vi "Destroy.vi"   [LabVIEW 2018, in "Toolkit.lvlib" / "Agent Identity.lvclass"]
doc: "Deallocates, or frees, the memory allocated for the agent identity object. After this is called, the object can no longer be used in the application without causing a segmentation fault, i.e. crashing LabVIEW. This VI must be called to avoid leaking memory or running out of memory on resource-constrained systems."
uses:
  Agent Identity.lvclass
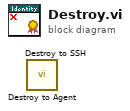
[diagram p0: block diagram]
diagram:
  n1 = call "Destroy to Agent.vi"() -> ()  [unwired: 10 in, 2 out]
  n2 = call "Destroy to SSH.vi"() -> ()  [unwired: 10 in, 2 out]
